vi "test-state-space-util.vi"(8 "error in (no error)":errorcluster) -> (0 "error out":errorcluster, 3 "All Tests Passed":bool)   [LabVIEW 2019]
uses:
  <vilib>/Analysis/Matrix/Datatypes/RealMatrix.ctl
  <vilib>/Rock Robotics/WPI/ThirdParty/JAS_Junk/TrajLib/MatBuilder_Create.vi
  <vilib>/Rock Robotics/WPI/ThirdParty/JAS_Junk/TrajLib/MatrixHelper_CoerceSize.vi
  <vilib>/Rock Robotics/WPI/ThirdParty/JAS_Junk/TrajLib/Rotation_CreateAngle.vi
  <vilib>/Rock Robotics/WPI/ThirdParty/JAS_Junk/TrajLib/Translation_Create.vi
  <vilib>/Analysis/7linalg.llb/Matrix Exp.vi
  <vilib>/Analysis/7linalg.llb/Real Matrix Exp.vi
  <vilib>/Rock Robotics/WPI/ThirdParty/JAS_Junk/TrajLib/Matrix_Transpose.vi
  <vilib>/Rock Robotics/WPI/ThirdParty/JAS_Junk/TrajLib/StateSpaceUtil_Check_Stabilizable.vi
  <vilib>/Utility/error.llb/Error Cluster From Error Code.vi
  <vilib>/Analysis/Matrix/Numeric/Multiply/Multiply - RM,R.vi
  <vilib>/Analysis/1siggen.llb/Gaussian White Noise.vi
  <vilib>/Rock Robotics/WPI/ThirdParty/JAS_Junk/TrajLib/Trajectory_Library.lvlib
  <vilib>/Analysis/Matrix/NI_Matrix.lvlib
  <vilib>/Analysis/NI_AALBase.lvlib
panel:
  out "standard deviation 2":dbl format="%0.2f"
  out "standard deviation":dbl format="%0.2f"
  out "exp test 1":bool
  out "exp test 0":bool
  out "is Detect Error 4":errorcluster
  out "is Detectable 4":bool
  out "is Detect Error 3":errorcluster
  out "is Detectable 3":bool
  out "is Detect Error 2":errorcluster
  out "is Detectable 2":bool
  out "is Detect Error 1":errorcluster
  out "is Detectable 1":bool
  out "Eigenvalues 4":cdb[](array[numeric])
  out "R rank 4":i32[](array[numeric])
  out "Error 4":errorcluster
  out "IsStabilizable 4":bool
  out "Eigenvalues 3":cdb[](array[numeric])
  out "R rank 3":i32[](array[numeric])
  out "Error 3":errorcluster
  out "IsStabilizable 3":bool
  out "Eigenvalues 2":cdb[](array[numeric])
  out "R rank 2":i32[](array[numeric])
  out "Error 2":errorcluster
  out "IsStabilizable 2":bool
  out "Eigenvalues":cdb[](array[numeric])
  out "R rank":i32[](array[numeric])
  out "Error":errorcluster
  out "IsStabilizable":bool
  out "Test Passed 1":bool
  out "Test Passed 0":bool
  out "Cost Mat 2":T1
  out "CoVar Mat 2":T1
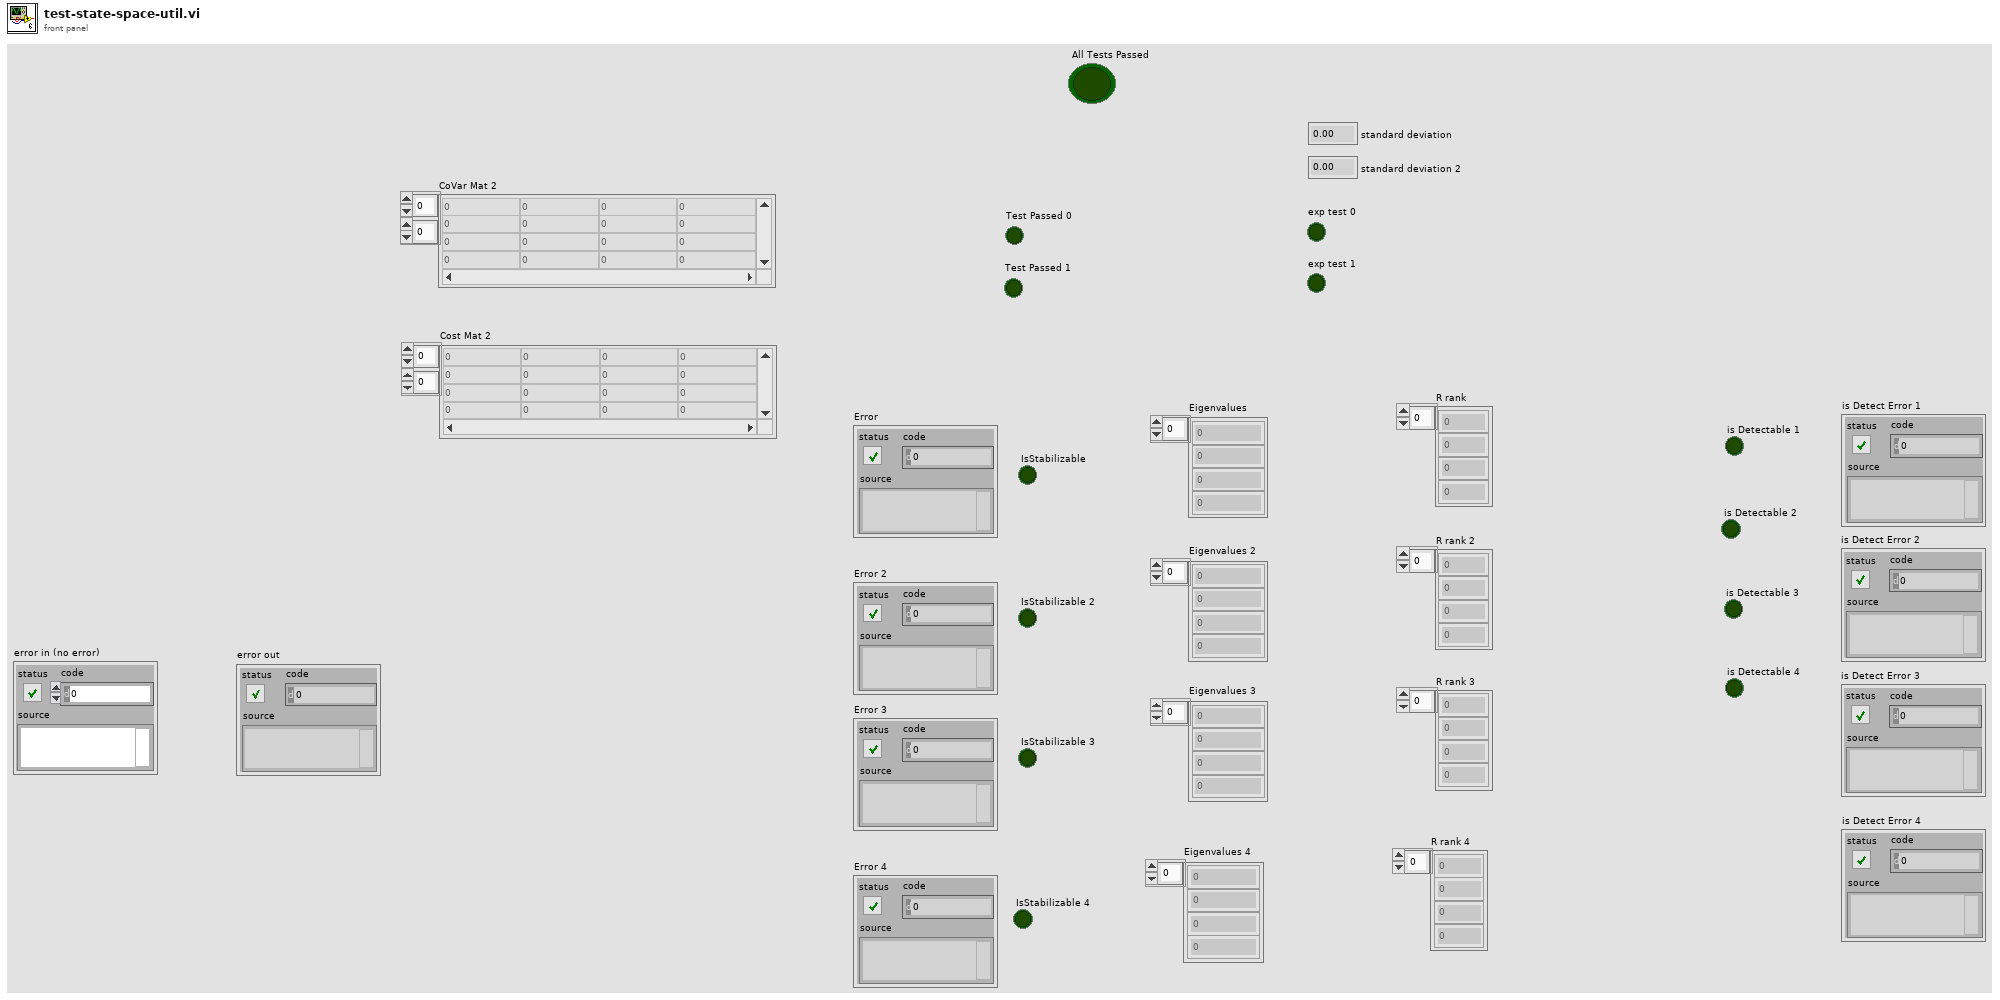
[diagram p1: front panel]
types:
  T1 = typedef "NI_Matrix.lvlib/RealMatrix.ctl" = dbl[][]
  T2 = typedef "Trajectory_Library.lvlib/POSE2D.ctl" = cluster{"TRANSLATION":T3, "ROTATION":T4}
  T3 = typedef "Trajectory_Library.lvlib/TRANSLATION2D.ctl" = cluster{"X":dbl, "Y":dbl}
  T4 = typedef "Trajectory_Library.lvlib/ROTATION2D.ctl" = cluster{"VALUE":dbl, "COS":dbl, "SIN":dbl}
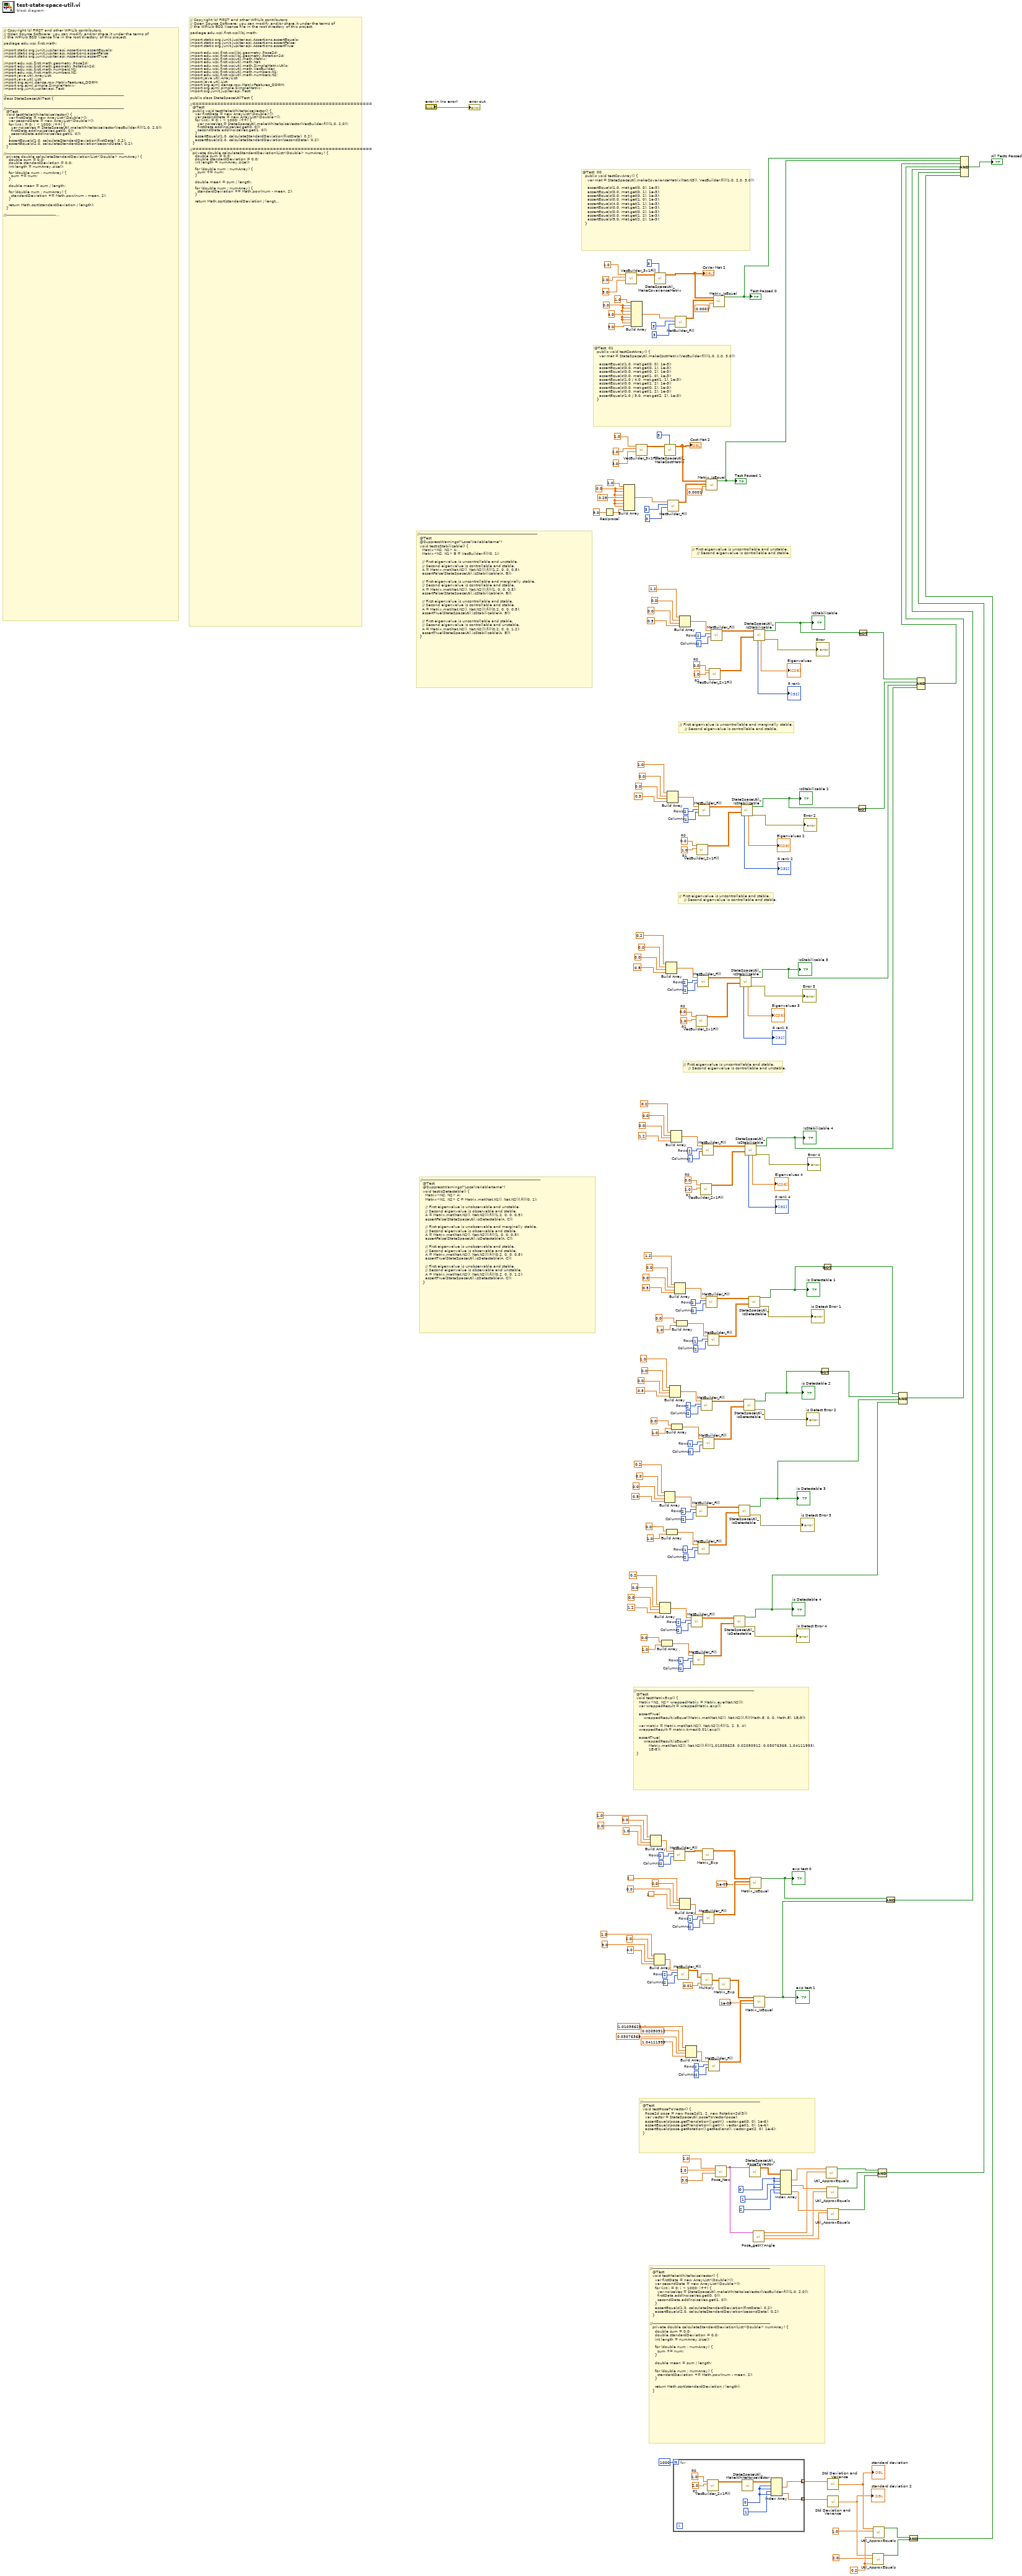
[diagram p0: block diagram]
diagram:
  w4 = 0.2 ("Tolerance")
  w25 = 0 ("index (row)")
  w43 = 2  # Columns
  w42 = 2  # Rows
  w48 = 2  # Columns
  w47 = 2  # Rows
  w59 = 2  # Columns
  w58 = 2  # Rows
  w65 = 2  # Columns
  w64 = 2  # Rows
  w92 = 2  # Columns
  w91 = 1  # Rows
  w98 = 2  # Columns
  w97 = 2  # Rows
  w106 = 2  # Columns
  w105 = 1  # Rows
  w112 = 2  # Columns
  w111 = 2  # Rows
  w120 = 2  # Columns
  w119 = 1  # Rows
  w126 = 2  # Columns
  w125 = 2  # Rows
  w134 = 2  # Columns
  w133 = 1  # Rows
  w140 = 2  # Columns
  w139 = 2  # Rows
  w157 = 1.0  # R1
  w156 = 0.0  # R0
  w159 = 2  # Columns
  w158 = 2  # Rows
  w169 = 1.0  # R1
  w168 = 0.0  # R0
  w171 = 2  # Columns
  w170 = 2  # Rows
  w181 = 1.0  # R1
  w180 = 0.0  # R0
  w183 = 2  # Columns
  w182 = 2  # Rows
  w193 = 1.0  # R1
  w192 = 0.0  # R0
  w195 = 2  # Columns
  w194 = 2  # Rows
  w209 = 0.0 ("element")
  w219 = 0.0 ("element")
  # "//-----------------------------------------------------------------------------------------------\n  @Test\n  void testMakeWhiteNoiseVector() {\n    var firstData = new ArrayList<Double>();\n    var secondData = new ArrayList<Double>();\n    for (int i = 0; i < 1000; i++) {\n      var noiseVec = StateSpaceUtil.makeWhiteNoiseVector(VecBuilder.fill(1.0, 2.0));\n      firstData.add(noiseVec.get(0, 0));\n      secondData.add(noiseVec.get(1, 0));\n    }\n    assertEquals(1.0, calculateStandardDeviation(firstData), 0.2);\n    assertEquals(2.0, calculateStandardDeviation(secondData), 0.2);\n  }\n\n//-----------------------------------------------------------------------------------------------\n  private double calculateStandardDeviation(List<Double> numArray) {\n    double sum = 0.0;\n    double standardDeviation = 0.0;\n    int length = numArray.size();\n\n    for (double num : numArray) {\n      sum += num;\n    }\n\n    double mean = sum / length;\n\n    for (double num : numArray) {\n      standardDeviation += Math.pow(num - mean, 2);\n    }\n\n    return Math.sqrt(standardDeviation / length);\n  }"
  # "//-----------------------------------------------------------------------------------------------\n  @Test\n  void testPoseToVector() {\n    Pose2d pose = new Pose2d(1, 2, new Rotation2d(3));\n    var vector = StateSpaceUtil.poseToVector(pose);\n    assertEquals(pose.getTranslation().getX(), vector.get(0, 0), 1e-6);\n    assertEquals(pose.getTranslation().getY(), vector.get(1, 0), 1e-6);\n    assertEquals(pose.getRotation().getRadians(), vector.get(2, 0), 1e-6);\n  }"
  # "//-----------------------------------------------------------------------------------------------\n  @Test\n  void testMatrixExp() {\n    Matrix<N2, N2> wrappedMatrix = Matrix.eye(Nat.N2());\n    var wrappedResult = wrappedMatrix.exp();\n\n    assertTrue(\n        wrappedResult.isEqual(Matrix.mat(Nat.N2(), Nat.N2()).fill(Math.E, 0, 0, Math.E), 1E-9));\n\n    var matrix = Matrix.mat(Nat.N2(), Nat.N2()).fill(1, 2, 3, 4);\n    wrappedResult = matrix.times(0.01).exp();\n\n    assertTrue(\n        wrappedResult.isEqual(\n            Matrix.mat(Nat.N2(), Nat.N2()).fill(1.01035625, 0.02050912, 0.03076368, 1.04111993),\n            1E-8));\n  }"
  # "//-----------------------------------------------------------------------------------------------\n  @Test\n  @SuppressWarnings(\"LocalVariableName\")\n  void testIsDetectable() {\n    Matrix<N2, N2> A;\n    Matrix<N1, N2> C = Matrix.mat(Nat.N1(), Nat.N2()).fill(0, 1);\n\n    // First eigenvalue is unobservable and unstable.\n    // Second eigenvalue is observable and stable.\n    A = Matrix.mat(Nat.N2(), Nat.N2()).fill(1.2, 0, 0, 0.5);\n    assertFalse(StateSpaceUtil.isDetectable(A, C));\n\n    // First eigenvalue is unobservable and marginally stable.\n    // Second eigenvalue is observable and stable.\n    A = Matrix.mat(Nat.N2(), Nat.N2()).fill(1, 0, 0, 0.5);\n    assertFalse(StateSpaceUtil.isDetectable(A, C));\n\n    // First eigenvalue is unobservable and stable.\n    // Second eigenvalue is observable and stable.\n    A = Matrix.mat(Nat.N2(), Nat.N2()).fill(0.2, 0, 0, 0.5);\n    assertTrue(StateSpaceUtil.isDetectable(A, C));\n\n    // First eigenvalue is unobservable and stable.\n    // Second eigenvalue is observable and unstable.\n    A = Matrix.mat(Nat.N2(), Nat.N2()).fill(0.2, 0, 0, 1.2);\n    assertTrue(StateSpaceUtil.isDetectable(A, C));\n  }"
  # "// First eigenvalue is uncontrollable and stable.\n    // Second eigenvalue is controllable and unstable."
  # "// First eigenvalue is uncontrollable and stable.\n    // Second eigenvalue is controllable and stable."
  # "// First eigenvalue is uncontrollable and marginally stable.\n    // Second eigenvalue is controllable and stable."
  # "// First eigenvalue is uncontrollable and unstable.\n    // Second eigenvalue is controllable and stable."
  # "//-----------------------------------------------------------------------------------------------\n  @Test\n  @SuppressWarnings(\"LocalVariableName\")\n  void testIsStabilizable() {\n    Matrix<N2, N2> A;\n    Matrix<N2, N1> B = VecBuilder.fill(0, 1);\n\n    // First eigenvalue is uncontrollable and unstable.\n    // Second eigenvalue is controllable and stable.\n    A = Matrix.mat(Nat.N2(), Nat.N2()).fill(1.2, 0, 0, 0.5);\n    assertFalse(StateSpaceUtil.isStabilizable(A, B));\n\n    // First eigenvalue is uncontrollable and marginally stable.\n    // Second eigenvalue is controllable and stable.\n    A = Matrix.mat(Nat.N2(), Nat.N2()).fill(1, 0, 0, 0.5);\n    assertFalse(StateSpaceUtil.isStabilizable(A, B));\n\n    // First eigenvalue is uncontrollable and stable.\n    // Second eigenvalue is controllable and stable.\n    A = Matrix.mat(Nat.N2(), Nat.N2()).fill(0.2, 0, 0, 0.5);\n    assertTrue(StateSpaceUtil.isStabilizable(A, B));\n\n    // First eigenvalue is uncontrollable and stable.\n    // Second eigenvalue is controllable and unstable.\n    A = Matrix.mat(Nat.N2(), Nat.N2()).fill(0.2, 0, 0, 1.2);\n    assertTrue(StateSpaceUtil.isStabilizable(A, B));\n  }"
  # "@Test  01\n  public void testCostArray() {\n    var mat = StateSpaceUtil.makeCostMatrix(VecBuilder.fill(1.0, 2.0, 3.0));\n\n    assertEquals(1.0, mat.get(0, 0), 1e-3);\n    assertEquals(0.0, mat.get(0, 1), 1e-3);\n    assertEquals(0.0, mat.get(0, 2), 1e-3);\n    assertEquals(0.0, mat.get(1, 0), 1e-3);\n    assertEquals(1.0 / 4.0, mat.get(1, 1), 1e-3);\n    assertEquals(0.0, mat.get(1, 2), 1e-3);\n    assertEquals(0.0, mat.get(0, 2), 1e-3);\n    assertEquals(0.0, mat.get(1, 2), 1e-3);\n    assertEquals(1.0 / 9.0, mat.get(2, 2), 1e-3);\n  }"
  # "@Test  00\n  public void testCovArray() {\n    var mat = StateSpaceUtil.makeCovarianceMatrix(Nat.N3(), VecBuilder.fill(1.0, 2.0, 3.0));\n\n    assertEquals(1.0, mat.get(0, 0), 1e-3);\n    assertEquals(0.0, mat.get(0, 1), 1e-3);\n    assertEquals(0.0, mat.get(0, 2), 1e-3);\n    assertEquals(0.0, mat.get(1, 0), 1e-3);\n    assertEquals(4.0, mat.get(1, 1), 1e-3);\n    assertEquals(0.0, mat.get(1, 2), 1e-3);\n    assertEquals(0.0, mat.get(0, 2), 1e-3);\n    assertEquals(0.0, mat.get(1, 2), 1e-3);\n    assertEquals(9.0, mat.get(2, 2), 1e-3);\n  }"
  # "// Copyright (c) FIRST and other WPILib contributors.\n// Open Source Software; you can modify and/or share it under the terms of\n// the WPILib BSD license file in the root directory of this project.\n\npackage edu.wpi.first.math;\n\nimport static org.junit.jupiter.api.Assertions.assertEquals;\nimport static org.junit.jupiter.api.Assertions.assertFalse;\nimport static org.junit.jupiter.api.Assertions.assertTrue;\n\nimport edu.wpi.first.math.geometry.Pose2d;\nimport edu.wpi.first.math.geometry.Rotation2d;\nimport edu.wpi.first.math.numbers.N1;\nimport edu.wpi.first.math.numbers.N2;\nimport java.util.ArrayList;\nimport java.util.List;\nimport org.ejml.dense.row.MatrixFeatures_DDRM;\nimport org.ejml.simple.SimpleMatrix;\nimport org.junit.jupiter.api.Test;\n\n//-----------------------------------------------------------------------------------------------\nclass StateSpaceUtilTest {\n\n\n//-----------------------------------------------------------------------------------------------\n  @Test\n  void testMakeWhiteNoiseVector() {\n    var firstData = new ArrayList<Double>();\n    var secondData = new ArrayList<Double>();\n    for (int i = 0; i < 1000; i++) {\n      var noiseVec = StateSpaceUtil.makeWhiteNoiseVector(VecBuilder.fill(1.0, 2.0));\n      firstData.add(noiseVec.get(0, 0));\n      secondData.add(noiseVec.get(1, 0));\n    }\n    assertEquals(1.0, calculateStandardDeviation(firstData), 0.2);\n    assertEquals(2.0, calculateStandardDeviation(secondData), 0.2);\n  }\n\n//-----------------------------------------------------------------------------------------------\n  private double calculateStandardDeviation(List<Double> numArray) {\n    double sum = 0.0;\n    double standardDeviation = 0.0;\n    int length = numArray.size();\n\n    for (double num : numArray) {\n      sum += num;\n    }\n\n    double mean = sum / length;\n\n    for (double num : numArray) {\n      standardDeviation += Math.pow(num - mean, 2);\n    }\n\n    return Math.sqrt(standardDeviation / length);\n  }\n\n//-----------------------------------------------------------------------------------------------\n  @Test\n  void testMatrixExp() {\n    Matrix<N2, N2> wrappedMatrix = Matrix.eye(Nat.N2());\n    var wrappedResult = wrappedMatrix.exp();\n\n    assertTrue(\n        wrappedResult.isEqual(Matrix.mat(Nat.N2(), Nat.N2()).fill(Math.E, 0, 0, Math.E), 1E-9));\n\n    var matrix = Matrix.mat(Nat.N2(), Nat.N2()).fill(1, 2, 3, 4);\n    wrappedResult = matrix.times(0.01).exp();\n\n    assertTrue(\n        wrappedResult.isEqual(\n            Matrix.mat(Nat.N2(), Nat.N2()).fill(1.01035625, 0.02050912, 0.03076368, 1.04111993),\n            1E-8));\n  }\n\n//-----------------------------------------------------------------------------------------------\n  @Test\n  void testSimpleMatrixExp() {\n    SimpleMatrix matrix = SimpleMatrixUtils.eye(2);\n    var result = SimpleMatrixUtils.exp(matrix);\n\n    assertTrue(\n        MatrixFeatures_DDRM.isIdentical(\n            result.getDDRM(),\n            new SimpleMatrix(2, 2, true, new double[] {Math.E, 0, 0, Math.E}).getDDRM(),\n            1E-9));\n\n    matrix = new SimpleMatrix(2, 2, true, new double[] {1, 2, 3, 4});\n    result = SimpleMatrixUtils.exp(matrix.scale(0.01));\n\n    assertTrue(\n        MatrixFeatures_DDRM.isIdentical(\n            result.getDDRM(),\n            new SimpleMatrix(\n                    2, 2, true, new double[] {1.01035625, 0.02050912, 0.03076368, 1.04111993})\n                .getDDRM(),\n            1E-8));\n  }\n\n//-----------------------------------------------------------------------------------------------\n  @Test\n  void testPoseToVector() {\n    Pose2d pose = new Pose2d(1, 2, new Rotation2d(3));\n    var vector = StateSpaceUtil.poseToVector(pose);\n    assertEquals(pose.getTranslation().getX(), vector.get(0, 0), 1e-6);\n    assertEquals(pose.getTranslation().getY(), vector.get(1, 0), 1e-6);\n    assertEquals(pose.getRotation().getRadians(), vector.get(2, 0), 1e-6);\n  }\n}"
  # "// Copyright (c) FIRST and other WPILib contributors.\n// Open Source Software; you can modify and/or share it under the terms of\n// the WPILib BSD license file in the root directory of this project.\n\npackage edu.wpi.first.wpilibj.math;\n\nimport static org.junit.jupiter.api.Assertions.assertEquals;\nimport static org.junit.jupiter.api.Assertions.assertFalse;\nimport static org.junit.jupiter.api.Assertions.assertTrue;\n\nimport edu.wpi.first.wpilibj.geometry.Pose2d;\nimport edu.wpi.first.wpilibj.geometry.Rotation2d;\nimport edu.wpi.first.wpiutil.math.Matrix;\nimport edu.wpi.first.wpiutil.math.Nat;\nimport edu.wpi.first.wpiutil.math.SimpleMatrixUtils;\nimport edu.wpi.first.wpiutil.math.VecBuilder;\nimport edu.wpi.first.wpiutil.math.numbers.N1;\nimport edu.wpi.first.wpiutil.math.numbers.N2;\nimport java.util.ArrayList;\nimport java.util.List;\nimport org.ejml.dense.row.MatrixFeatures_DDRM;\nimport org.ejml.simple.SimpleMatrix;\nimport org.junit.jupiter.api.Test;\n\npublic class StateSpaceUtilTest {\n\n//==========================================================\n  @Test\n  public void testMakeWhiteNoiseVector() {\n    var firstData = new ArrayList<Double>();\n    var secondData = new ArrayList<Double>();\n    for (int i = 0; i < 1000; i++) {\n      var noiseVec = StateSpaceUtil.makeWhiteNoiseVector(VecBuilder.fill(1.0, 2.0));\n      firstData.add(noiseVec.get(0, 0));\n      secondData.add(noiseVec.get(1, 0));\n    }\n    assertEquals(1.0, calculateStandardDeviation(firstData), 0.2);\n    assertEquals(2.0, calculateStandardDeviation(secondData), 0.2);\n  }\n\n//==========================================================\n  private double calculateStandardDeviation(List<Double> numArray) {\n    double sum = 0.0;\n    double standardDeviation = 0.0;\n    int length = numArray.size();\n\n    for (double num : numArray) {\n      sum += num;\n    }\n\n    double mean = sum / length;\n\n    for (double num : numArray) {\n      standardDeviation += Math.pow(num - mean, 2);\n    }\n\n    return Math.sqrt(standardDeviation / length);\n  }\n\n\n//==========================================================\n    @Test\n  public void testMatrixExp() {\n    Matrix<N2, N2> wrappedMatrix = Matrix.eye(Nat.N2());\n    var wrappedResult = wrappedMatrix.exp();\n\n    assertTrue(\n        wrappedResult.isEqual(Matrix.mat(Nat.N2(), Nat.N2()).fill(Math.E, 0, 0, Math.E), 1E-9));\n\n    var matrix = Matrix.mat(Nat.N2(), Nat.N2()).fill(1, 2, 3, 4);\n    wrappedResult = matrix.times(0.01).exp();\n\n    assertTrue(\n        wrappedResult.isEqual(\n            Matrix.mat(Nat.N2(), Nat.N2()).fill(1.01035625, 0.02050912, 0.03076368, 1.04111993),\n            1E-8));\n  }\n\n//==========================================================\n  @Test\n  public void testSimpleMatrixExp() {\n    SimpleMatrix matrix = SimpleMatrixUtils.eye(2);\n    var result = SimpleMatrixUtils.exp(matrix);\n\n    assertTrue(\n        MatrixFeatures_DDRM.isIdentical(\n            result.getDDRM(),\n            new SimpleMatrix(2, 2, true, new double[] {Math.E, 0, 0, Math.E}).getDDRM(),\n            1E-9));\n\n    matrix = new SimpleMatrix(2, 2, true, new double[] {1, 2, 3, 4});\n    result = SimpleMatrixUtils.exp(matrix.scale(0.01));\n\n    assertTrue(\n        MatrixFeatures_DDRM.isIdentical(\n            result.getDDRM(),\n            new SimpleMatrix(\n                    2, 2, true, new double[] {1.01035625, 0.02050912, 0.03076368, 1.04111993})\n                .getDDRM(),\n            1E-8));\n  }\n\n//==========================================================\n  @Test\n  public void testPoseToVector() {\n    Pose2d pose = new Pose2d(1, 2, new Rotation2d(3));\n    var vector = StateSpaceUtil.poseToVector(pose);\n    assertEquals(pose.getTranslation().getX(), vector.get(0, 0), 1e-6);\n    assertEquals(pose.getTranslation().getY(), vector.get(1, 0), 1e-6);\n    assertEquals(pose.getRotation().getRadians(), vector.get(2, 0), 1e-6);\n  }\n}"
  n1 = Reciprocal(x=9.0 ("element")) -> (1/x=w205:dbl)
  n2 = Build Array(1.0 ("element"), w209, w209, w209, 0.25 ("element"), w209, w209, w209, w205) -> (w212:dbl[])
  n3 = call <vilib>:"VecBuilder_3x1Fill.vi"("R2"=3.0, "R1"=2.0, "R0"=1.0) -> ("output matrix"=w231:T1)  [unwired: 8 in]
  n4 = Build Array(1.0 ("element"), w219, w219, w219, 4.0 ("element"), w219, w219, w219, 9.0 ("element")) -> (w222:dbl[])
  n5 = call <vilib>:"VecBuilder_3x1Fill.vi"("R2"=3.0, "R1"=2.0, "R0"=1.0) -> ("output matrix"=w226:T1)  [unwired: 8 in]
  n6 = Build Array(1.0 ("element"), 0.0 ("element"), 0.0 ("element"), 1.0 ("element")) -> (w70:dbl[])
  n7 = Build Array(1.0 ("element"), 2.0 ("element"), 3.0 ("element"), 4.0 ("element")) -> (w53:dbl[])
  n8 = call <vilib>:"StateSpaceUtil_MakeCovarianceMatrix.vi"("States"=3, "StdDevs"=w231) -> ("Covariance Matrix"=w217:T1)  [unwired: 8 in, 1 out]
  "CoVar Mat 2" <- w217
  n9 = Build Array(0.2 ("element"), 0.0 ("element"), 0.0 ("element"), 1.2 ("element")) -> (w103:dbl[])
  n10 = Build Array(0.0 ("element"), 1.0 ("element")) -> (w95:dbl[])
  n11 = Build Array(0.2 ("element"), 0.0 ("element"), 0.0 ("element"), 0.5 ("element")) -> (w117:dbl[])
  n12 = call <vilib>:"StateSpaceUtil_MakeCostMatrix.vi"("States"=3, "Costs"=w226) -> ("Costs Matrix"=w204:T1)  [unwired: 8 in, 1 out]
  "Cost Mat 2" <- w204
  n13 = Build Array(0.2 ("element"), 0.0 ("element"), 0.0 ("element"), 0.5 ("element")) -> (w176:dbl[])
  n14 = Build Array(0.0 ("element"), 1.0 ("element")) -> (w109:dbl[])
  n15 = Build Array(1.0 ("element"), 0.0 ("element"), 0.0 ("element"), 0.5 ("element")) -> (w188:dbl[])
  n16 = call <vilib>:"MatBuilder_Fill.vi"("Columns"=3, "Rows"=3, "Value List"=w212) -> ("output matrix"=w208:T1)  [unwired: 8 in]
  n17 = Build Array(1.0 ("element"), 0.0 ("element"), 0.0 ("element"), 0.5 ("element")) -> (w131:dbl[])
  n18 = Build Array(0.2 ("element"), 0.0 ("element"), 0.0 ("element"), 1.2 ("element")) -> (w164:dbl[])
  n19 = Build Array(0.0 ("element"), 1.0 ("element")) -> (w123:dbl[])
  n20 = for {
    N: 1000 -> [_]
    tunnel: [w237] -> w9 mode=indexing
    tunnel: [w236] -> w10 mode=indexing
    w240 = 0 ("index (row)")
    w243 = 2.0  # R1
    w242 = 1.0  # R0
    n21 = call <vilib>:"VecBuilder_2x1Fill.vi"("R1"=w243, "R0"=w242) -> ("output matrix"=w241:T1)  [unwired: 9 in]
    n22 = call <vilib>:"StateSpaceUtil_MakeWhiteNoiseVector.vi"("StdDevs"=w241) -> ("WhiteNoise"=w238:T1)  [unwired: 9 in, 1 out]
    n23 = Index Array(array=w238, index (row) #1=w240, index (col) #1=w240, index (row) #2=1 ("index (row)"), index (col) #2=w240) -> (element #1=w237:dbl, element #2=w236:dbl)
  }
  n24 = call <vilib>:"MatBuilder_Fill.vi"("Columns"=w65, "Rows"=w64, "Value List"=w70) -> ("output matrix"=w63:T1)  [unwired: 8 in]
  n25 = Build Array(1.2 ("element"), 0.0 ("element"), 0.0 ("element"), 0.5 ("element")) -> (w145:dbl[])
  n26 = call <vilib>:"MatBuilder_Fill.vi"("Columns"=3, "Rows"=3, "Value List"=w222) -> ("output matrix"=w216:T1)  [unwired: 8 in]
  n27 = Build Array(0.0 ("element"), 1.0 ("element")) -> (w137:dbl[])
  n28 = call <vilib>:"MatBuilder_Fill.vi"("Columns"=w48, "Rows"=w47, "Value List"=w53) -> ("output matrix"=w38:T1)  [unwired: 8 in]
  n29 = Build Array(1.2 ("element"), 0.0 ("element"), 0.0 ("element"), 0.5 ("element")) -> (w200:dbl[])
  n30 = Build Array(2.718281828459045, 0.0 ("element"), 0.0 ("element"), 2.718281828459045) -> (w62:dbl[])
  n31 = Build Array(1.01035625 ("element"), 0.02050912 ("element"), 0.03076368 ("element"), 1.04111993 ("element")) -> (w46:dbl[])
  n32 = call <vilib>:"MatBuilder_Fill.vi"("Columns"=w98, "Rows"=w97, "Value List"=w103) -> ("output matrix"=w96:T1)  [unwired: 8 in]
  n33 = call <vilib>:"MatBuilder_Fill.vi"("Columns"=w92, "Rows"=w91, "Value List"=w95) -> ("output matrix"=w90:T1)  [unwired: 8 in]
  n34 = call <vilib>:"VecBuilder_2x1Fill.vi"("R1"=w169, "R0"=w168) -> ("output matrix"=w166:T1)  [unwired: 9 in]
  n35 = call <vilib>:"MatBuilder_Fill.vi"("Columns"=w112, "Rows"=w111, "Value List"=w117) -> ("output matrix"=w110:T1)  [unwired: 8 in]
  n36 = call <vilib>:"VecBuilder_2x1Fill.vi"("R1"=w181, "R0"=w180) -> ("output matrix"=w178:T1)  [unwired: 9 in]
  n37 = call <vilib>:"MatBuilder_Fill.vi"("Columns"=w171, "Rows"=w170, "Value List"=w176) -> ("output matrix"=w167:T1)  [unwired: 8 in]
  n38 = call <vilib>:"MatBuilder_Fill.vi"("Columns"=w106, "Rows"=w105, "Value List"=w109) -> ("output matrix"=w104:T1)  [unwired: 8 in]
  n39 = call <vilib>:"MatBuilder_Fill.vi"("Columns"=w183, "Rows"=w182, "Value List"=w188) -> ("output matrix"=w179:T1)  [unwired: 8 in]
  n40 = call <vilib>:"VecBuilder_2x1Fill.vi"("R1"=w157, "R0"=w156) -> ("output matrix"=w154:T1)  [unwired: 9 in]
  n41 = call <vilib>:"MatBuilder_Fill.vi"("Columns"=w126, "Rows"=w125, "Value List"=w131) -> ("output matrix"=w124:T1)  [unwired: 8 in]
  n42 = call-poly <vilib>:"Multiply.vi"("Real Scalar c"=0.01 ("y"), "Real Matrix A"=w38) -> ("A * c"=w37:T1)
  n43 = call <vilib>:"MatBuilder_Fill.vi"("Columns"=w159, "Rows"=w158, "Value List"=w164) -> ("output matrix"=w155:T1)  [unwired: 8 in]
  n44 = call <vilib>:"Matrix_Exp.vi"("input matrix"=w63) -> ("output matrix"=w55:T1)  [unwired: 9 in, 1 out]
  n45 = call <vilib>:"MatBuilder_Fill.vi"("Columns"=w120, "Rows"=w119, "Value List"=w123) -> ("output matrix"=w118:T1)  [unwired: 8 in]
  n46 = call <vilib>:"MatBuilder_Fill.vi"("Columns"=w59, "Rows"=w58, "Value List"=w62) -> ("output matrix"=w54:T1)  [unwired: 8 in]
  n47 = call <vilib>:"MatBuilder_Fill.vi"("Columns"=w140, "Rows"=w139, "Value List"=w145) -> ("output matrix"=w138:T1)  [unwired: 8 in]
  n48 = call <vilib>:"Matrix_IsEqual.vi"("Tolerance"=0.0001, "other"=w208, "input matrix"=w204) -> ("Equal"=w201:bool)  [unwired: 8 in]
  "Test Passed 1" <- w201
  n49 = call <vilib>:"MatBuilder_Fill.vi"("Columns"=w134, "Rows"=w133, "Value List"=w137) -> ("output matrix"=w132:T1)  [unwired: 8 in]
  n50 = call <vilib>:"MatBuilder_Fill.vi"("Columns"=w43, "Rows"=w42, "Value List"=w46) -> ("output matrix"=w40:T1)  [unwired: 8 in]
  n51 = call <vilib>:"VecBuilder_2x1Fill.vi"("R1"=w193, "R0"=w192) -> ("output matrix"=w190:T1)  [unwired: 9 in]
  n52 = call <vilib>:"MatBuilder_Fill.vi"("Columns"=w195, "Rows"=w194, "Value List"=w200) -> ("output matrix"=w191:T1)  [unwired: 8 in]
  n53 = call <vilib>:"Matrix_IsEqual.vi"("Tolerance"=0.0001, "other"=w216, "input matrix"=w217) -> ("Equal"=w202:bool)  [unwired: 8 in]
  "Test Passed 0" <- w202
  n54 = call <vilib>:"Pose_New.vi"("Heading"=3.0 ("Angle"), "Y"=2.0, "X"=1.0) -> ("out POSe"=w19:T2)  [unwired: 8 in]
  n55 = call <vilib>:"Matrix_Exp.vi"("input matrix"=w37) -> ("output matrix"=w41:T1)  [unwired: 9 in, 1 out]
  n56 = call <vilib>:"StateSpaceUtil_IsDetectable.vi"("C"=w90, "A"=w96) -> ("Error"=→"is Detect Error 4":errorcluster, "IsDetectable"=w72:bool)  [unwired: 8 in]
  "is Detectable 4" <- w72
  n57 = call <vilib>:"StateSpaceUtil_IsDetectable.vi"("C"=w104, "A"=w110) -> ("Error"=→"is Detect Error 3":errorcluster, "IsDetectable"=w73:bool)  [unwired: 8 in]
  "is Detectable 3" <- w73
  n58 = call <vilib>:"StateSpaceUtil_IsStabilizable.vi"("B"=w166, "A"=w167) -> ("Error"=→"Error 3":errorcluster, "IsStabilizable"=w148:bool, "Eigenvalues"=→"Eigenvalues 3":cdb[], "R rank"=→"R rank 3":i32[])  [unwired: 6 in]
  "IsStabilizable 3" <- w148
  n59 = call <vilib>:"StateSpaceUtil_IsStabilizable.vi"("B"=w178, "A"=w179) -> ("Error"=→"Error 2":errorcluster, "IsStabilizable"=w151:bool, "Eigenvalues"=→"Eigenvalues 2":cdb[], "R rank"=→"R rank 2":i32[])  [unwired: 6 in]
  "IsStabilizable 2" <- w151
  n60 = call <vilib>:"StateSpaceUtil_IsDetectable.vi"("C"=w118, "A"=w124) -> ("Error"=→"is Detect Error 2":errorcluster, "IsDetectable"=w75:bool)  [unwired: 8 in]
  "is Detectable 2" <- w75
  n61 = call <vilib>:"StateSpaceUtil_IsStabilizable.vi"("B"=w154, "A"=w155) -> ("Error"=→"Error 4":errorcluster, "IsStabilizable"=w147:bool, "Eigenvalues"=→"Eigenvalues 4":cdb[], "R rank"=→"R rank 4":i32[])  [unwired: 6 in]
  "IsStabilizable 4" <- w147
  n62 = call <vilib>:"StateSpaceUtil_IsDetectable.vi"("C"=w132, "A"=w138) -> ("Error"=→"is Detect Error 1":errorcluster, "IsDetectable"=w76:bool)  [unwired: 8 in]
  "is Detectable 1" <- w76
  n63 = call <vilib>:"StateSpaceUtil_PoseToVector.vi"("Pose"=w19) -> ("Pose Vector"=w26:T1)  [unwired: 10 in]
  n64 = call <vilib>:"Matrix_IsEqual.vi"("Tolerance"=1e-09, "other"=w54, "input matrix"=w55) -> ("Equal"=w32:bool)  [unwired: 8 in]
  "exp test 0" <- w32
  n65 = call <vilib>:"Pose_getXYAngle.vi"("in POSE"=w19) -> ("Angle"=w16:dbl, "Y"=w17:dbl, "X"=w18:dbl)  [unwired: 8 in]
  n66 = call <vilib>:"StateSpaceUtil_IsStabilizable.vi"("B"=w190, "A"=w191) -> ("Error"=→"Error":errorcluster, "IsStabilizable"=w152:bool, "Eigenvalues"=→"Eigenvalues":cdb[], "R rank"=→"R rank":i32[])  [unwired: 6 in]
  "IsStabilizable" <- w152
  n67 = call <vilib>:"Matrix_IsEqual.vi"("Tolerance"=1e-08, "other"=w40, "input matrix"=w41) -> ("Equal"=w31:bool)  [unwired: 8 in]
  "exp test 1" <- w31
  n68 = Index Array(array=w26, index (row) #1=w25, index (col) #1=w25, index (row) #2=1 ("index (row)"), index (col) #2=w25, index (row) #3=2 ("index (row)"), index (col) #3=w25) -> (element #1=w22:dbl, element #2=w21:dbl, element #3=w20:dbl)
  n69 = Not(x=w75) -> (.not. x?=w74:bool)
  n70 = Not(x=w76) -> (.not. x?=w77:bool)
  n71 = call <vilib>:"Util_ApproxEquals.vi"("Value 2"=w18, "Value 1"=w22) -> ("ApproxEquals"=w15:bool)  [unwired: 9 in]
  n72 = call <vilib>:"Util_ApproxEquals.vi"("Value 2"=w17, "Value 1"=w21) -> ("ApproxEquals"=w14:bool)  [unwired: 9 in]
  n73 = call <vilib>:"Util_ApproxEquals.vi"("Value 2"=w16, "Value 1"=w20) -> ("ApproxEquals"=w13:bool)  [unwired: 9 in]
  n74 = call <vilib>:"Std Deviation and Variance.vi"("X"=w9) -> ("standard deviation"=w8:dbl)  [unwired: 1 in, 2 out]
  "standard deviation" <- w8
  n75 = call <vilib>:"Std Deviation and Variance.vi"("X"=w10) -> ("standard deviation"=w7:dbl)  [unwired: 1 in, 2 out]
  "standard deviation 2" <- w7
  n76 = Not(x=w151) -> (.not. x?=w149:bool)
  n77 = Not(x=w152) -> (.not. x?=w150:bool)
  n78 = call <vilib>:"Util_ApproxEquals.vi"("Tolerance"=w4, "Value 2"=2.0, "Value 1"=w7) -> ("ApproxEquals"=w2:bool)  [unwired: 8 in]
  n79 = call <vilib>:"Util_ApproxEquals.vi"("Tolerance"=w4, "Value 2"=1.0, "Value 1"=w8) -> ("ApproxEquals"=w3:bool)  [unwired: 8 in]
  n80 = Compound Arithmetic op=AND(w15, w14, w13) -> (w12:bool)
  n81 = Compound Arithmetic op=AND(w32, w31) -> (w30:bool)
  n82 = Compound Arithmetic op=AND(w77, w74, w73, w72) -> (w71:bool)
  n83 = And(x=w3, y=w2) -> (x .and. y?=w1:bool)
  n84 = Compound Arithmetic op=AND(w150, w149, w148, w147) -> (w146:bool)
  n85 = Compound Arithmetic op=AND(w202, w201, w146, w71, w30, w12, w1) -> (→"All Tests Passed":bool)
  "error out" <- "error in (no error)"
